vi "Untitled 2.vi"() -> ()   [LabVIEW 2026]
panel:
  out "first":dbl format="%#_6p"
  out "second":dbl format="%#_6p"
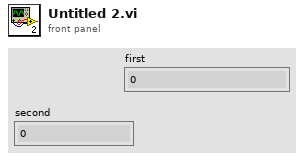
[diagram p1: front panel]
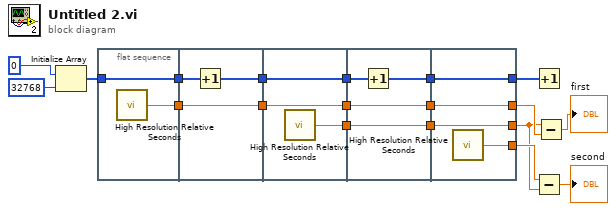
[diagram p0: block diagram]
diagram:
  n1 = Initialize Array(u8 0 ("element"), 32768 ("dimension size")) -> (w17:u8[])
  n2 = flat-sequence {
    tunnel: w17 -> [w21]
    tunnel: [w21] -> w16
    tunnel: [w20] -> w15
    tunnel: w16 -> [w24]
    tunnel: w15 -> [w23]
    tunnel: [w23] -> w14
    tunnel: [w22] -> w12
    tunnel: w14 -> [w26]
    tunnel: w12 -> [w25]
    tunnel: [w27] -> w11
    tunnel: [w26] -> w10
    tunnel: [w25] -> w9
    tunnel: w11 -> [w31]
    tunnel: w10 -> [w30]
    tunnel: w9 -> [w29]
    tunnel: [w31] -> w8
    tunnel: [w30] -> w7
    tunnel: [w28] -> w2
    tunnel: [w34] -> w13
    tunnel: [w35] -> w5
    tunnel: w8 -> [w35]
    tunnel: w7 -> [w34]
    tunnel: [w33] -> w6
    tunnel: [w32] -> w1
    tunnel: w2 -> [w32]
    frame #0 {
      n3 = call <vilib>:"High Resolution Relative Seconds.vi"() -> ("relative seconds"=w20:dbl)
    }
    frame #1 {
      n4 = Increment(x=w24) -> (x+1=w22:u8[])
    }
    frame #2 {
      n5 = call <vilib>:"High Resolution Relative Seconds.vi"() -> ("relative seconds"=w27:dbl)
    }
    frame #3 {
      n6 = Increment(x=w29) -> (x+1=w28:u8[])
    }
    frame #4 {
      n7 = call <vilib>:"High Resolution Relative Seconds.vi"() -> ("relative seconds"=w33:dbl)
    }
  }
  n8 = Increment(x=w1) -> ()  [unwired: 1 out]
  n9 = Subtract(x=w6, y=w5) -> (x-y=→"second":dbl)
  n10 = Subtract(x=w5, y=w13) -> (x-y=→"first":dbl)
